vi "Begin.vi"() -> (0 "error out":errorcluster)   [LabVIEW 2013]
doc: "Called before other user functions, this VI is expected to open initial I/O refnums, load in file data, and do all program initialization. Notice that the <B>error out</B> terminal is simply used for data flow. Wiring it to other structures or subVIs ensures that this VI runs first."
uses:
  <vilib>/Rock Robotics/WPI/DriverStation/WPI_DriverStationRobotMode2.ctl
  <vilib>/Rock Robotics/SystemInterfaces/DIO/FPGA_DIOChannel.ctl
  <vilib>/Rock Robotics/SystemInterfaces/DIO/FPGA_DIORelayChannel.ctl
  <vilib>/Rock Robotics/SystemInterfaces/DIO/FPGA_DIOPWMChannel.ctl
  <vilib>/Rock Robotics/WPI/SafetyOutput/WPI_SafetyOutputConfigMenu.ctl
  <vilib>/Rock Robotics/WPI/Relay/WPI_RelayDirection.ctl
  <vilib>/Rock Robotics/WPI/Joystick/WPI_JoystickDeviceEnum.ctl
  <vilib>/Rock Robotics/WPI/Solenoid/WPI_SolenoidChannel.ctl
  <vilib>/Rock Robotics/WPI/Solenoid/WPI_SolenoidValue.ctl
  <vilib>/Rock Robotics/SystemInterfaces/CounterEncoderSourceConvertion/FPGA_CounterEncoderSourceConvertionLVSourceType.ctl
  <vilib>/Rock Robotics/SystemInterfaces/Typedef/FPGA_TypedefDigitalModule.ctl
  <vilib>/Rock Robotics/SystemInterfaces/DIO/FPGA_DIODigitalSourceChannel.ctl
  <vilib>/Rock Robotics/SystemInterfaces/AnalogTrigger/FPGA_AnalogTriggerIndex.ctl
  <vilib>/Rock Robotics/SystemInterfaces/AnalogTrigger/FPGA_AnalogTriggerOutType.ctl
  Robot Global Data.vi
  <vilib>/Rock Robotics/WPI/RobotDrive/WPI_RobotDriveOpen4MotorWithJaguar.vi
  <vilib>/Rock Robotics/WPI/MotorControl/WPI_MotorControlOpen Jaguar.vi
  <vilib>/Rock Robotics/WPI/Solenoid/WPI_SolenoidOpenDouble.vi
  <vilib>/Rock Robotics/WPI/Solenoid/WPI_SolenoidSetEnum.vi
  <vilib>/Rock Robotics/WPI/Compressor/WPI_CompressorGetSetRefNum.vi
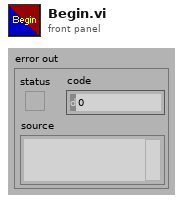
[diagram p1: front panel]
types:
  T1 = enum16{"ToPos2", "ToPos1", "Fire", "Wait", "ESTOP", "Reset", "ToLowPower", "ToHighPower"}
  T2 = typedef "FPGA_DIORelayChannel.ctl" = enum8{"Relay 1", "Relay 2", "Relay 3", "Relay 4", "Relay 5", "Relay 6", "Relay 7", "Relay 8", "Invalid"}
  T3 = typedef "FPGA_DIOChannel.ctl" = enum8{"DIO 1", "DIO 2", "DIO 3", "DIO 4", "DIO 5", "DIO 6", "DIO 7", "DIO 8", "DIO 9", "DIO 10", "DIO 11", "DIO 12", "DIO 13", "DIO 14", "Invalid"}
  T4 = typedef "WPI_DriverStationRobotMode2.ctl" = enum16{"Autonomous Disabled", "Autonomous Enabled", "Teleop Disabled", "Teleop Enabled", "Timeout", "Finish", "Test Disabled", "Test Enabled"}
  T5 = typedef "FPGA_DIOPWMChannel.ctl" = enum8{"PWM 1", "PWM 2", "PWM 3", "PWM 4", "PWM 5", "PWM 6", "PWM 7", "PWM 8", "PWM 9", "PWM 10", "Invalid"}
  T6 = typedef "WPI_SafetyOutputConfigMenu.ctl" = enum16{"Enable", "Disable"}
  T7 = typedef "WPI_MotorControlDeviceRef.ctl" = cluster{"DeviceStatus":errorcluster, "Type":enum16{"PWM", "CAN"}, "PWM":cluster{"Digital Module":T8, "PWM Channel":T5, "DeadBand":T9}, "CAN":cluster{"Device Number":u8, "Control Mode":T10, "Semaphore":T11, "Max Vout":dbl}, "Invert":bool, "TransformRef":T12, "InvTransformRef":T12}
  T8 = typedef "FPGA_TypedefDigitalModule.ctl" = enum16{"Digital Module 1", "Digital Module 2"}
  T9 = typedef "WPI_PWMDeadband.ctl" = cluster{"Name":string, "maxPositivePwm":i32, "minPositivePwm":i32, "centerPwm":i32, "maxNegativePwm":i32, "minNegativePwm":i32, "angularRange":u16}
  T10 = typedef "WPI_CANJaguar_ControlMode.ctl" = enum8{"Percent VBus", "Current", "Speed", "Position", "Voltage"}
  T11 = typedef "Semaphore RefNum" = refnum<k1>
  T12 = typedef "WPI_PWMTransform_ConPane.ctl" = refnum<vi>
  T13 = typedef "WPI_RobotDriveDevRef.ctl" = cluster{"DevStatus":errorcluster, "Motors[]":T7[], "Square Inputs":bool, "Max Output":dbl, "Isochronous":bool}
  T14 = typedef "FPGA_CounterEncoderSourceConvertionLVSourceType.ctl" = cluster{"DevStatus":errorcluster, "AnalogTriggerMode?":bool, "DigitalMode":cluster{"Digital Module":T8, "DIO Channel":T15}, "AnalogTriggerMode":cluster{"AnalogTriggerIndex":T16, "OutputType":T17}}
  T15 = typedef "FPGA_DIODigitalSourceChannel.ctl" = enum8{"DIO 1", "DIO 2", "DIO 3", "DIO 4", "DIO 5", "DIO 6", "DIO 7", "DIO 8", "DIO 9", "DIO 10", "DIO 11", "DIO 12", "DIO 13", "DIO 14", "Disabled"}
  T16 = typedef "FPGA_AnalogTriggerIndex.ctl" = enum8{"Trig 0", "Trig 1", "Trig 2", "Trig 3", "Trig 4", "Trig 5", "Trig 6", "Trig 7", "Invalid"}
  T17 = typedef "FPGA_AnalogTriggerOutType.ctl" = enum16{"InWindow", "TriggerState", "Rising", "Falling"}
  T18 = typedef "WPI_EncoderDevRef.ctl" = cluster{"DevStatus":errorcluster, "EncoderIndex":T19, "CounterIndex":T20, "DistancePerCount":dbl, "Decoding Type":T21}
  T19 = typedef "FPGA_EncoderIdx.ctl" = enum8{"Enc 0", "Enc 1", "Enc 2", "Enc 3", "Invalid"}
  T20 = typedef "FPGA_CounterCtrSystemIndex.ctl" = enum8{"Ctr 0", "Ctr 1", "Ctr 2", "Ctr 3", "Ctr 4", "Ctr 5", "Ctr 6", "Ctr 7", "Invalid"}
  T21 = typedef "WPI_EncoderType.ctl" = enum16{"1x", "2x", "4x"}
  T22 = typedef "WPI_SolenoidValue.ctl" = enum16{"Off", "On", "Forward", "Reverse"}
  T23 = typedef "WPI_SolenoidChannel.ctl" = enum8{"Solenoid 1", "Solenoid 2", "Solenoid 3", "Solenoid 4", "Solenoid 5", "Solenoid 6", "Solenoid 7", "Solenoid 8", "Invalid"}
  T24 = typedef "WPI_SolenoidDevRef.ctl" = cluster{"DevStatus":errorcluster, "Solenoid Module":T25, "Forward Solenoid Channel":T23, "Reverse Solenoid Channel":T23}
  T25 = typedef "FPGA_TypedefSolenoidModule.ctl" = enum16{"Solenoid Module 1", "Solenoid Module 2"}
  T26 = typedef "WPI_RelayDirection.ctl" = enum16{"Both directions", "Forward only", "Reverse only"}
  T27 = typedef "WPI_RelayDevRef.ctl" = cluster{"DevStatus":errorcluster, "Relay Channel":T2, "Digital Module":T8, "Relay Direction":T26}
  T28 = typedef "WPI_DigitalInputDevRef.ctl" = cluster{"DevStatus":errorcluster, "DIO Channel":T3, "Digital Module":T8}
  T29 = typedef "WPI_JoystickDeviceEnum.ctl" = enum16{"USB 1", "USB 2", "USB 3", "USB 4", "Kinect 1", "Kinect 2"}
  T30 = typedef "WPI_JoystickDevRef.ctl" = cluster{"Device":T29}
  T31 = typedef "WPI_CompressorDevRef.ctl" = cluster{"DevStatus":errorcluster, "DigitalInputDevRef":T28, "RelayDevRef":T27}
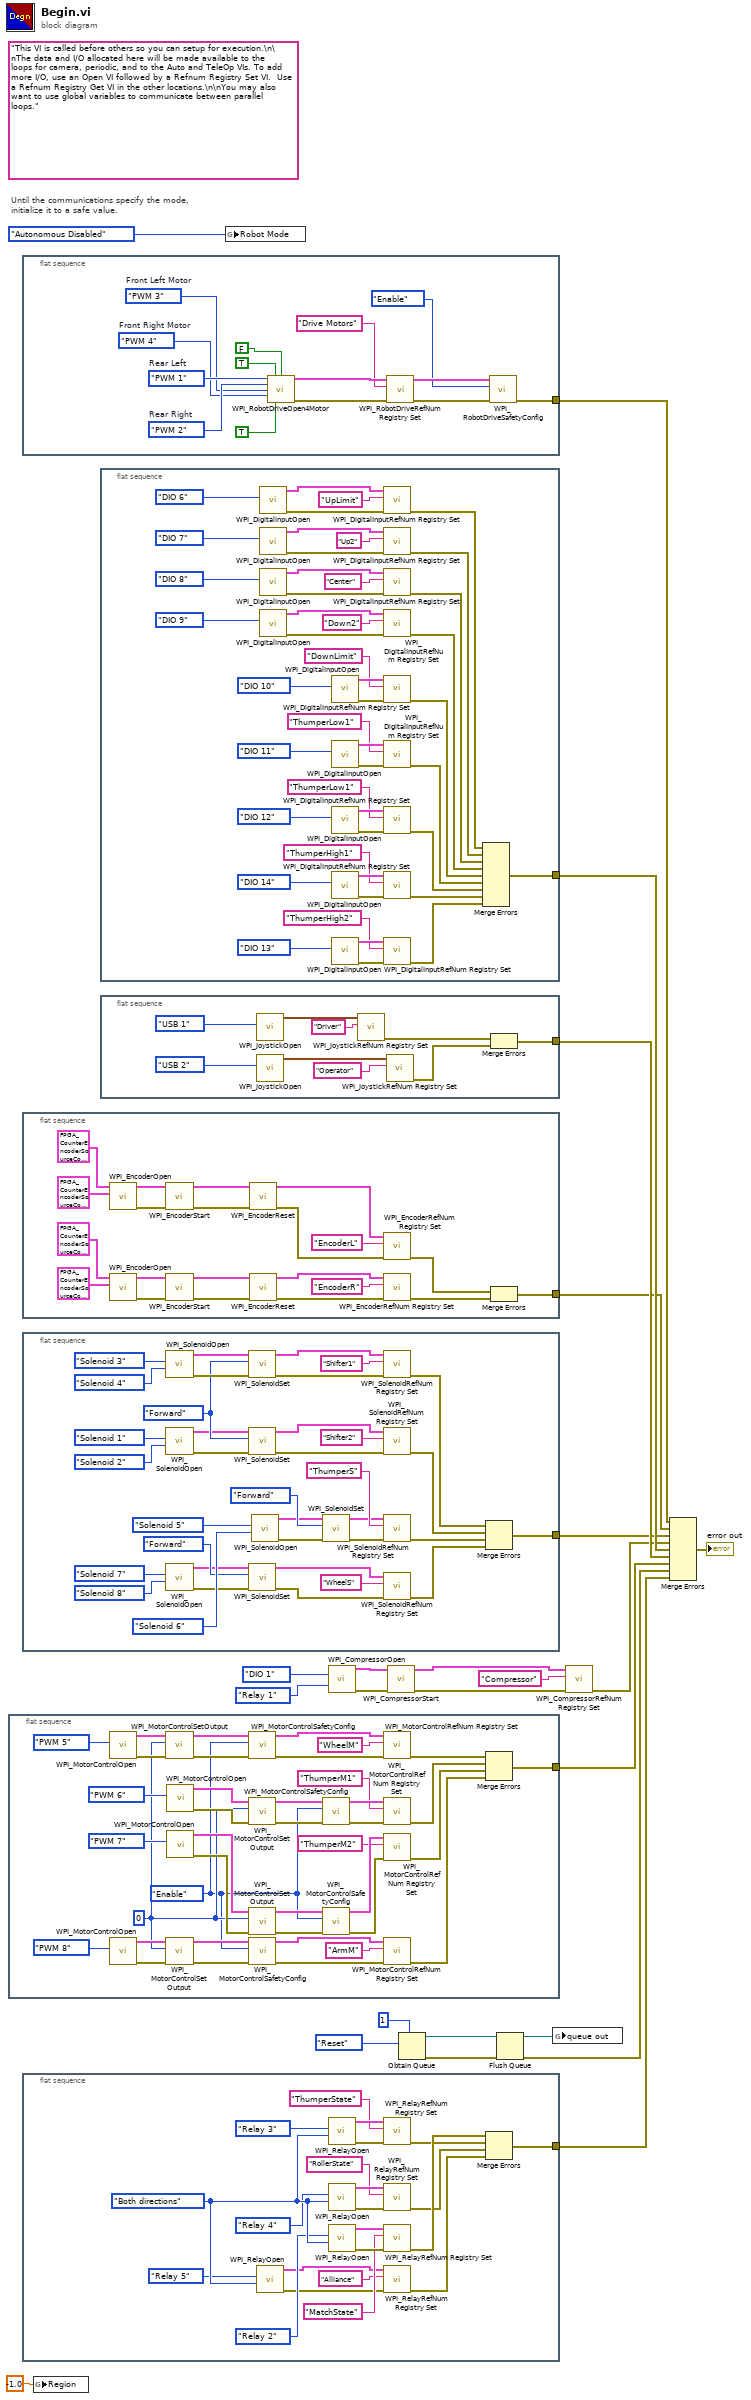
[diagram p0: block diagram]
diagram:
  (unwired) "This VI is called before others so you can setup for execution.\n\nThe data and I/O allocated here will be made available to the loops for camera, periodic, and to the Auto and TeleOp VIs. To add more I/O, use an Open VI followed by a Refnum Registry Set VI.  Use a Refnum Registry Get VI in the other locations.\n\nYou may also want to use global variables to communicate between parallel loops."
  # "Until the communications specify the mode,\ninitialize it to a safe value."
  n1 = flat-sequence {
    tunnel: [w25] -> w11
    frame #0 {
      w30 = WPI_SafetyOutputConfigMenu."Enable" ("mode")
      w31 = 0
      n2 = call-poly <vilib>:"WPI_MotorControlOpen.vi"("PWM Channel"=FPGA_DIOPWMChannel."PWM 5") -> ("error out"=w58:errorcluster, "MotorControlDeviceRef"=w59:T7)  [unwired: 9 in]
      n3 = call-poly <vilib>:"WPI_MotorControlOpen.vi"("PWM Channel"=FPGA_DIOPWMChannel."PWM 8") -> ("error out"=w56:errorcluster, "MotorControlDeviceRef"=w57:T7)  [unwired: 9 in]
      n4 = call <vilib>:"WPI_MotorControlSetOutput.vi"("error in (no error)"=w58, "Output"=w31, "MotorControlDevRef"=w59) -> ("error out"=w40:errorcluster, "MotorControlDevRef"=w41:T7)  [unwired: 6 in, 1 out]
      n5 = call <vilib>:"WPI_MotorControlSetOutput.vi"("error in (no error)"=w56, "Output"=w31, "MotorControlDevRef"=w57) -> ("error out"=w38:errorcluster, "MotorControlDevRef"=w39:T7)  [unwired: 6 in, 1 out]
      n6 = call-poly <vilib>:"WPI_MotorControlOpen.vi"("PWM Channel"=FPGA_DIOPWMChannel."PWM 6") -> ("error out"=w52:errorcluster, "MotorControlDeviceRef"=w53:T7)  [unwired: 9 in]
      n7 = call-poly <vilib>:"WPI_MotorControlOpen.vi"("PWM Channel"=FPGA_DIOPWMChannel."PWM 7") -> ("error out"=w55:errorcluster, "MotorControlDeviceRef"=w54:T7)  [unwired: 9 in]
      n8 = call <vilib>:"WPI_MotorControlSafetyConfig.vi"("error in (no error)"=w40, "mode"=w30, "MotorControlDevRef"=w41) -> ("error out"=w48:errorcluster, "MotorControlDevRef"=w49:T7)  [unwired: 7 in]
      n9 = call <vilib>:"WPI_MotorControlSetOutput.vi"("error in (no error)"=w52, "Output"=w31, "MotorControlDevRef"=w53) -> ("error out"=w36:errorcluster, "MotorControlDevRef"=w37:T7)  [unwired: 6 in, 1 out]
      n10 = call <vilib>:"WPI_MotorControlSetOutput.vi"("error in (no error)"=w55, "Output"=w31, "MotorControlDevRef"=w54) -> ("error out"=w42:errorcluster, "MotorControlDevRef"=w43:T7)  [unwired: 6 in, 1 out]
      n11 = call <vilib>:"WPI_MotorControlSafetyConfig.vi"("error in (no error)"=w38, "mode"=w30, "MotorControlDevRef"=w39) -> ("error out"=w44:errorcluster, "MotorControlDevRef"=w45:T7)  [unwired: 7 in]
      n12 = call <vilib>:"WPI_MotorControlSafetyConfig.vi"("error in (no error)"=w36, "mode"=w30, "MotorControlDevRef"=w37) -> ("error out"=w50:errorcluster, "MotorControlDevRef"=w51:T7)  [unwired: 7 in]
      n13 = call <vilib>:"WPI_MotorControlSafetyConfig.vi"("error in (no error)"=w42, "mode"=w30, "MotorControlDevRef"=w43) -> ("error out"=w46:errorcluster, "MotorControlDevRef"=w47:T7)  [unwired: 7 in]
      n14 = call <vilib>:"WPI_MotorControlRefNum Registry Set.vi"("error in (no error)"=w48, "refnum name"="WheelM", "MotorControlDevRef"=w49) -> ("error out"=w29:errorcluster)  [unwired: 7 in, 1 out]
      n15 = call <vilib>:"WPI_MotorControlRefNum Registry Set.vi"("error in (no error)"=w50, "refnum name"="ThumperM1", "MotorControlDevRef"=w51) -> ("error out"=w28:errorcluster)  [unwired: 7 in, 1 out]
      n16 = call <vilib>:"WPI_MotorControlRefNum Registry Set.vi"("error in (no error)"=w46, "refnum name"="ThumperM2", "MotorControlDevRef"=w47) -> ("error out"=w27:errorcluster)  [unwired: 7 in, 1 out]
      n17 = call <vilib>:"WPI_MotorControlRefNum Registry Set.vi"("error in (no error)"=w44, "refnum name"="ArmM", "MotorControlDevRef"=w45) -> ("error out"=w26:errorcluster)  [unwired: 7 in, 1 out]
      n18 = Merge Errors(w29, w28, w27, w26) -> (w25:errorcluster)
    }
  }
  n19 = flat-sequence {
    tunnel: [w77] -> w6
    frame #0 {
      w66 = FPGA_DIOPWMChannel."PWM 4"  # Front Right Motor
      w67 = FPGA_DIOPWMChannel."PWM 3"  # Front Left Motor
      w70 = FPGA_DIOPWMChannel."PWM 2"  # Rear Right
      w71 = FPGA_DIOPWMChannel."PWM 1"  # Rear Left
      n20 = call-poly <vilib>:"WPI_RobotDriveOpen4Motor.vi"("Rear Left Motor"=w71, "Rear Left Motor Inverted"=TRUE ("LeftMotorInverted"), "Rear Right Motor Inverted"=FALSE ("RightMotorInverted"), "Rear Right Motor"=w70, "Front Left Motor"=w67, "Front Right Motor"=w66, "Front Left Motor Inverted"=TRUE) -> ("RobotDriveDevRef"=w74:T13, "error out"=w72:errorcluster)  [unwired: 7 in]
      n21 = call <vilib>:"WPI_RobotDriveRefNum Registry Set.vi"("error in (no error)"=w72, "refnum name"="Drive Motors", "RobotDriveDevRef"=w74) -> ("error out"=w64:errorcluster, "RobotDriveDevRef"=w69:T13)  [unwired: 7 out]
      n22 = call <vilib>:"WPI_RobotDriveSafetyConfig.vi"("error in (no error)"=w64, "mode"=WPI_SafetyOutputConfigMenu."Enable", "RobotDriveDevRef"=w69) -> ("error out"=w77:errorcluster)  [unwired: 7 in, 1 out]
    }
  }
  n23 = flat-sequence {
    tunnel: [w78] -> w5
    frame #0 {
      n24 = call <vilib>:"WPI_EncoderOpen.vi"("BSource"=T14 {"DevStatus"={"status"=FALSE, "code"=0, "source"=""}, "AnalogTriggerMode?"=FALSE, "DigitalMode"={"Digital Module"=enum."Digital Module 1", "DIO Channel"=enum."DIO 3"}, "AnalogTriggerMode"={"AnalogTriggerIndex"=enum."Trig 0", "OutputType"=enum."InWindow"}} ("BSource 2"), "ASource"=T14 {"DevStatus"={"status"=FALSE, "code"=0, "source"=""}, "AnalogTriggerMode?"=FALSE, "DigitalMode"={"Digital Module"=enum."Digital Module 1", "DIO Channel"=enum."DIO 2"}, "AnalogTriggerMode"={"AnalogTriggerIndex"=enum."Trig 0", "OutputType"=enum."InWindow"}} ("ASource 2")) -> ("error out"=w81:errorcluster, "EncoderDevRef"=w82:T18)  [unwired: 8 in]
      n25 = call <vilib>:"WPI_EncoderOpen.vi"("BSource"=T14 {"DevStatus"={"status"=FALSE, "code"=0, "source"=""}, "AnalogTriggerMode?"=FALSE, "DigitalMode"={"Digital Module"=enum."Digital Module 1", "DIO Channel"=enum."DIO 5"}, "AnalogTriggerMode"={"AnalogTriggerIndex"=enum."Trig 0", "OutputType"=enum."InWindow"}}, "ASource"=T14 {"DevStatus"={"status"=FALSE, "code"=0, "source"=""}, "AnalogTriggerMode?"=FALSE, "DigitalMode"={"Digital Module"=enum."Digital Module 1", "DIO Channel"=enum."DIO 4"}, "AnalogTriggerMode"={"AnalogTriggerIndex"=enum."Trig 0", "OutputType"=enum."InWindow"}}) -> ("error out"=w90:errorcluster, "EncoderDevRef"=w91:T18)  [unwired: 8 in]
      n26 = call <vilib>:"WPI_EncoderStart.vi"("error in (no error)"=w81, "EncoderDevRef"=w82) -> ("error out"=w83:errorcluster, "EncoderDevRef"=w84:T18)  [unwired: 8 in]
      n27 = call <vilib>:"WPI_EncoderStart.vi"("error in (no error)"=w90, "EncoderDevRef"=w91) -> ("error out"=w92:errorcluster, "EncoderDevRef"=w93:T18)  [unwired: 8 in]
      n28 = call <vilib>:"WPI_EncoderReset.vi"("error in (no error)"=w83, "EncoderDevRef"=w84) -> ("error out"=w85:errorcluster, "EncoderDevRef"=w86:T18)  [unwired: 8 in]
      n29 = call <vilib>:"WPI_EncoderReset.vi"("error in (no error)"=w92, "EncoderDevRef"=w93) -> ("error out"=w94:errorcluster, "EncoderDevRef"=w95:T18)  [unwired: 8 in]
      n30 = call <vilib>:"WPI_EncoderRefNum Registry Set.vi"("error in (no error)"=w85, "refnum name"="EncoderL", "EncoderDevRef"=w86) -> ("error out"=w80:errorcluster)  [unwired: 7 in, 1 out]
      n31 = call <vilib>:"WPI_EncoderRefNum Registry Set.vi"("error in (no error)"=w94, "refnum name"="EncoderR", "EncoderDevRef"=w95) -> ("error out"=w79:errorcluster)  [unwired: 7 in, 1 out]
      n32 = Merge Errors(w80, w79) -> (w78:errorcluster)
    }
  }
  n33 = flat-sequence {
    tunnel: [w99] -> w7
    frame #0 {
      w126 = WPI_SolenoidValue."Forward" ("Value")
      n34 = call-poly <vilib>:"WPI_SolenoidOpen.vi"("Reverse Solenoid Channel"=WPI_SolenoidChannel."Solenoid 4", "Forward Solenoid Channel"=WPI_SolenoidChannel."Solenoid 3") -> ("error out"=w131:errorcluster, "SolenoidDevRef"=w130:T24)  [unwired: 8 in]
      n35 = call-poly <vilib>:"WPI_SolenoidOpen.vi"("Reverse Solenoid Channel"=WPI_SolenoidChannel."Solenoid 2", "Forward Solenoid Channel"=WPI_SolenoidChannel."Solenoid 1") -> ("error out"=w123:errorcluster, "SolenoidDevRef"=w122:T24)  [unwired: 8 in]
      n36 = call-poly <vilib>:"WPI_SolenoidOpen.vi"("Reverse Solenoid Channel"=WPI_SolenoidChannel."Solenoid 8", "Forward Solenoid Channel"=WPI_SolenoidChannel."Solenoid 7") -> ("error out"=w106:errorcluster, "SolenoidDevRef"=w107:T24)  [unwired: 8 in]
      n37 = call-poly <vilib>:"WPI_SolenoidSet.vi"("error in (no error)"=w131, "Value"=w126, "SolenoidDevRef"=w130) -> ("error out"=w132:errorcluster, "SolenoidDevRef"=w133:T24)  [unwired: 7 in]
      n38 = call-poly <vilib>:"WPI_SolenoidSet.vi"("error in (no error)"=w123, "Value"=w126, "SolenoidDevRef"=w122) -> ("error out"=w125:errorcluster, "SolenoidDevRef"=w124:T24)  [unwired: 7 in]
      n39 = call-poly <vilib>:"WPI_SolenoidSet.vi"("error in (no error)"=w106, "Value"=WPI_SolenoidValue."Forward", "SolenoidDevRef"=w107) -> ("error out"=w109:errorcluster, "SolenoidDevRef"=w110:T24)  [unwired: 7 in]
      n40 = call-poly <vilib>:"WPI_SolenoidOpen.vi"("Reverse Solenoid Channel"=WPI_SolenoidChannel."Solenoid 6", "Forward Solenoid Channel"=WPI_SolenoidChannel."Solenoid 5" ("Solenoid Channel")) -> ("error out"=w114:errorcluster, "SolenoidDevRef"=w115:T24)  [unwired: 8 in]
      n41 = call-poly <vilib>:"WPI_SolenoidSet.vi"("error in (no error)"=w114, "Value"=WPI_SolenoidValue."Forward", "SolenoidDevRef"=w115) -> ("error out"=w117:errorcluster, "SolenoidDevRef"=w118:T24)  [unwired: 7 in]
      n42 = call <vilib>:"WPI_SolenoidRefNum Registry Set.vi"("error in (no error)"=w132, "refnum name"="Shifter1", "SolenoidDevRef"=w133) -> ("error out"=w103:errorcluster)  [unwired: 7 in, 1 out]
      n43 = call <vilib>:"WPI_SolenoidRefNum Registry Set.vi"("error in (no error)"=w125, "refnum name"="Shifter2", "SolenoidDevRef"=w124) -> ("error out"=w102:errorcluster)  [unwired: 7 in, 1 out]
      n44 = call <vilib>:"WPI_SolenoidRefNum Registry Set.vi"("error in (no error)"=w117, "refnum name"="ThumperS", "SolenoidDevRef"=w118) -> ("error out"=w101:errorcluster)  [unwired: 7 in, 1 out]
      n45 = call <vilib>:"WPI_SolenoidRefNum Registry Set.vi"("error in (no error)"=w109, "refnum name"="WheelS", "SolenoidDevRef"=w110) -> ("error out"=w100:errorcluster)  [unwired: 7 in, 1 out]
      n46 = Merge Errors(w103, w102, w101, w100) -> (w99:errorcluster)
    }
  }
  n47 = flat-sequence {
    tunnel: [w135] -> w1
    frame #0 {
      w156 = WPI_RelayDirection."Both directions" ("Relay Direction")
      n48 = call <vilib>:"WPI_RelayOpen.vi"("Relay Direction"=w156, "Relay Channel"=FPGA_DIORelayChannel."Relay 5") -> ("error out"=w142:errorcluster, "RelayDevRef"=w143:T27)  [unwired: 8 in]
      n49 = call <vilib>:"WPI_RelayOpen.vi"("Relay Direction"=w156, "Relay Channel"=FPGA_DIORelayChannel."Relay 3") -> ("error out"=w149:errorcluster, "RelayDevRef"=w150:T27)  [unwired: 8 in]
      n50 = call <vilib>:"WPI_RelayOpen.vi"("Relay Direction"=w156, "Relay Channel"=FPGA_DIORelayChannel."Relay 4") -> ("error out"=w145:errorcluster, "RelayDevRef"=w146:T27)  [unwired: 8 in]
      n51 = call <vilib>:"WPI_RelayOpen.vi"("Relay Direction"=w156, "Relay Channel"=FPGA_DIORelayChannel."Relay 2") -> ("error out"=w154:errorcluster, "RelayDevRef"=w155:T27)  [unwired: 8 in]
      n52 = call <vilib>:"WPI_RelayRefNum Registry Set.vi"("error in (no error)"=w149, "refnum name"="ThumperState", "RelayDevRef"=w150) -> ("error out"=w138:errorcluster)  [unwired: 7 in, 1 out]
      n53 = call <vilib>:"WPI_RelayRefNum Registry Set.vi"("error in (no error)"=w145, "refnum name"="RollerState", "RelayDevRef"=w146) -> ("error out"=w137:errorcluster)  [unwired: 7 in, 1 out]
      n54 = call <vilib>:"WPI_RelayRefNum Registry Set.vi"("error in (no error)"=w154, "refnum name"="MatchState", "RelayDevRef"=w155) -> ("error out"=w139:errorcluster)  [unwired: 7 in, 1 out]
      n55 = call <vilib>:"WPI_RelayRefNum Registry Set.vi"("error in (no error)"=w142, "refnum name"="Alliance", "RelayDevRef"=w143) -> ("error out"=w136:errorcluster)  [unwired: 7 in, 1 out]
      n56 = Merge Errors(w139, w138, w137, w136) -> (w135:errorcluster)
    }
  }
  n57 = global write "Robot Global Data.vi" "Region"(-1.0 ("Region")) -> ()
  n58 = flat-sequence {
    tunnel: [w157] -> w10
    frame #0 {
      n59 = call <vilib>:"WPI_DigitalInputOpen.vi"("DIO Channel"=FPGA_DIOChannel."DIO 6") -> ("error out"=w196:errorcluster, "DigitalInputDevRef"=w197:T28)  [unwired: 9 in]
      n60 = call <vilib>:"WPI_DigitalInputOpen.vi"("DIO Channel"=FPGA_DIOChannel."DIO 7") -> ("error out"=w181:errorcluster, "DigitalInputDevRef"=w180:T28)  [unwired: 9 in]
      n61 = call <vilib>:"WPI_DigitalInputOpen.vi"("DIO Channel"=FPGA_DIOChannel."DIO 8") -> ("error out"=w185:errorcluster, "DigitalInputDevRef"=w184:T28)  [unwired: 9 in]
      n62 = call <vilib>:"WPI_DigitalInputOpen.vi"("DIO Channel"=FPGA_DIOChannel."DIO 9") -> ("error out"=w183:errorcluster, "DigitalInputDevRef"=w182:T28)  [unwired: 9 in]
      n63 = call <vilib>:"WPI_DigitalInputOpen.vi"("DIO Channel"=FPGA_DIOChannel."DIO 10") -> ("error out"=w202:errorcluster, "DigitalInputDevRef"=w201:T28)  [unwired: 9 in]
      n64 = call <vilib>:"WPI_DigitalInputOpen.vi"("DIO Channel"=FPGA_DIOChannel."DIO 11") -> ("error out"=w169:errorcluster, "DigitalInputDevRef"=w168:T28)  [unwired: 9 in]
      n65 = call <vilib>:"WPI_DigitalInputOpen.vi"("DIO Channel"=FPGA_DIOChannel."DIO 12") -> ("error out"=w189:errorcluster, "DigitalInputDevRef"=w188:T28)  [unwired: 9 in]
      n66 = call <vilib>:"WPI_DigitalInputOpen.vi"("DIO Channel"=FPGA_DIOChannel."DIO 14") -> ("error out"=w187:errorcluster, "DigitalInputDevRef"=w186:T28)  [unwired: 9 in]
      n67 = call <vilib>:"WPI_DigitalInputOpen.vi"("DIO Channel"=FPGA_DIOChannel."DIO 13") -> ("error out"=w172:errorcluster, "DigitalInputDevRef"=w171:T28)  [unwired: 9 in]
      n68 = call <vilib>:"WPI_DigitalInputRefNum Registry Set.vi"("error in (no error)"=w196, "refnum name"="UpLimit", "DigitalInputDevRef"=w197) -> ("error out"=w166:errorcluster)  [unwired: 7 in, 1 out]
      n69 = call <vilib>:"WPI_DigitalInputRefNum Registry Set.vi"("error in (no error)"=w181, "refnum name"="Up2", "DigitalInputDevRef"=w180) -> ("error out"=w165:errorcluster)  [unwired: 7 in, 1 out]
      n70 = call <vilib>:"WPI_DigitalInputRefNum Registry Set.vi"("error in (no error)"=w185, "refnum name"="Center", "DigitalInputDevRef"=w184) -> ("error out"=w164:errorcluster)  [unwired: 7 in, 1 out]
      n71 = call <vilib>:"WPI_DigitalInputRefNum Registry Set.vi"("error in (no error)"=w183, "refnum name"="Down2", "DigitalInputDevRef"=w182) -> ("error out"=w163:errorcluster)  [unwired: 7 in, 1 out]
      n72 = call <vilib>:"WPI_DigitalInputRefNum Registry Set.vi"("error in (no error)"=w202, "refnum name"="DownLimit", "DigitalInputDevRef"=w201) -> ("error out"=w162:errorcluster)  [unwired: 7 in, 1 out]
      n73 = call <vilib>:"WPI_DigitalInputRefNum Registry Set.vi"("error in (no error)"=w169, "refnum name"="ThumperLow1", "DigitalInputDevRef"=w168) -> ("error out"=w161:errorcluster)  [unwired: 7 in, 1 out]
      n74 = call <vilib>:"WPI_DigitalInputRefNum Registry Set.vi"("error in (no error)"=w189, "refnum name"="ThumperLow1", "DigitalInputDevRef"=w188) -> ("error out"=w160:errorcluster)  [unwired: 7 in, 1 out]
      n75 = call <vilib>:"WPI_DigitalInputRefNum Registry Set.vi"("error in (no error)"=w187, "refnum name"="ThumperHigh1", "DigitalInputDevRef"=w186) -> ("error out"=w159:errorcluster)  [unwired: 7 in, 1 out]
      n76 = call <vilib>:"WPI_DigitalInputRefNum Registry Set.vi"("error in (no error)"=w172, "refnum name"="ThumperHigh2", "DigitalInputDevRef"=w171) -> ("error out"=w158:errorcluster)  [unwired: 7 in, 1 out]
      n77 = Merge Errors(w166, w165, w164, w163, w162, w161, w160, w159, w158) -> (w157:errorcluster)
    }
  }
  n78 = flat-sequence {
    tunnel: [w203] -> w9
    frame #0 {
      n79 = call <vilib>:"WPI_JoystickOpen.vi"("JoystickDevice"=WPI_JoystickDeviceEnum."USB 1") -> ("JoystickDevRef"=w207:T30)  [unwired: 10 in]
      n80 = call <vilib>:"WPI_JoystickOpen.vi"("JoystickDevice"=WPI_JoystickDeviceEnum."USB 2") -> ("JoystickDevRef"=w210:T30)  [unwired: 10 in]
      n81 = call <vilib>:"WPI_JoystickRefNum Registry Set.vi"("refnum name"="Driver", "JoystickDevRef"=w207) -> ("error out"=w205:errorcluster)  [unwired: 8 in, 1 out]
      n82 = call <vilib>:"WPI_JoystickRefNum Registry Set.vi"("refnum name"="Operator", "JoystickDevRef"=w210) -> ("error out"=w204:errorcluster)  [unwired: 8 in, 1 out]
      n83 = Merge Errors(w205, w204) -> (w203:errorcluster)
    }
  }
  n84 = global write "Robot Global Data.vi" "Robot Mode"(WPI_DriverStationRobotMode2."Autonomous Disabled" ("Robot Mode")) -> ()
  n85 = call <vilib>:"WPI_CompressorOpen.vi"("Pressure Switch DIO Channel"=FPGA_DIOChannel."DIO 1", "Relay Channel"=FPGA_DIORelayChannel."Relay 1") -> ("CompressorDevRef"=w20:T31, "error out"=w19:errorcluster)  [unwired: 12 in]
  n86 = call <vilib>:"WPI_CompressorStart.vi"("error in (no error)"=w19, "CompressorDevRef"=w20) -> ("error out"=w18:errorcluster, "CompressorDevRef"=w17:T31)  [unwired: 8 in]
  n87 = Obtain Queue(max queue size (-1, unlimited)=1, element data type=T1."Reset" ("element")) -> (queue out=w14:refnum<queue>, error out=w15:errorcluster)  [unwired: 3 in, 1 out]
  n88 = Flush Queue(queue=w14, error in (no error)=w15) -> (queue out=w3:refnum<queue>, error out=w12:errorcluster)  [unwired: 1 out]
  n89 = global write "Robot Global Data.vi" "queue out"(w3) -> ()
  n90 = call <vilib>:"WPI_CompressorRefNum Registry Set.vi"("error in (no error)"=w18, "refnum name"="Compressor", "CompressorDevRef"=w17) -> ("error out"=w8:errorcluster)  [unwired: 7 in, 1 out]
  n91 = Merge Errors(w6, w5, w7, w8, w10, w9, w11, w12, w1) -> (→"error out":errorcluster)
